vi "主流程.vi"() -> ()   [LabVIEW 2016]
panel:
  out "通讯包字符串":string
  out "列表选择":T1(ring)
  out "枚举":T2(ring)
  out "数据输出":string
  in  "IP":string
  in  "远程端口或服务名称":u16
  in  "停止 2":bool
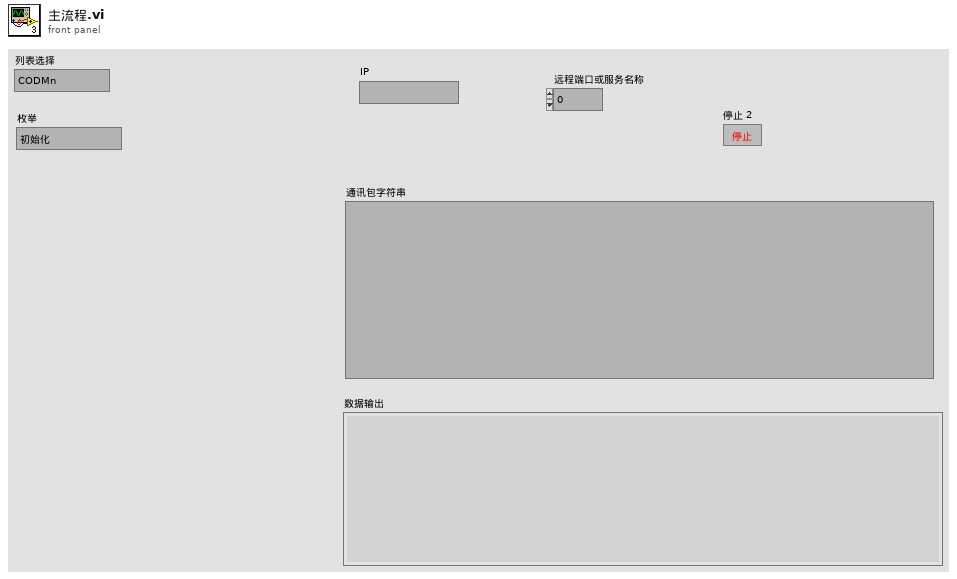
[diagram p1: front panel]
types:
  T1 = enum16{"CODMn", "CODMn空白核查", "CODMn标样核查", "氨氮", "氨氮空白核查", "氨氮标样核查", "多参数", "多参标样核查", "总磷", "总磷空白核查", "总磷标样核查", "总氮", "总氮空白核查", "总氮标样核查"}
  T2 = enum16{"初始化", "打开连接", "表格比对", "发送数据", "读取数据", "数据发送成功", "数据发送失败"}
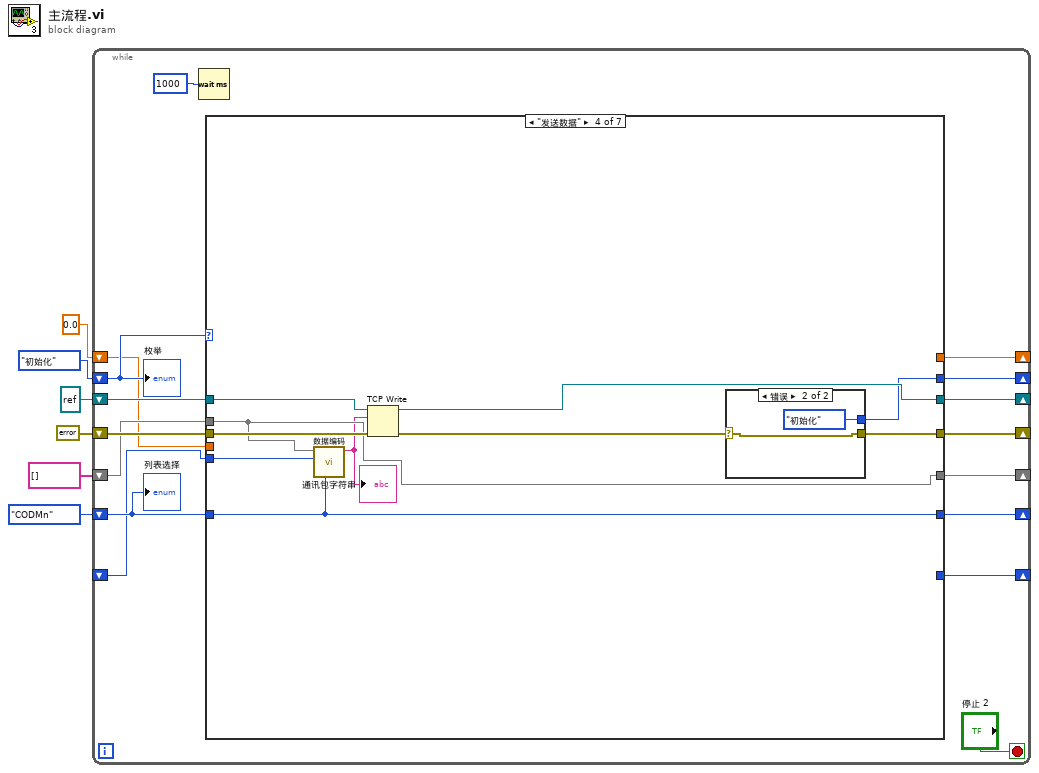
[diagram p0: block diagram]
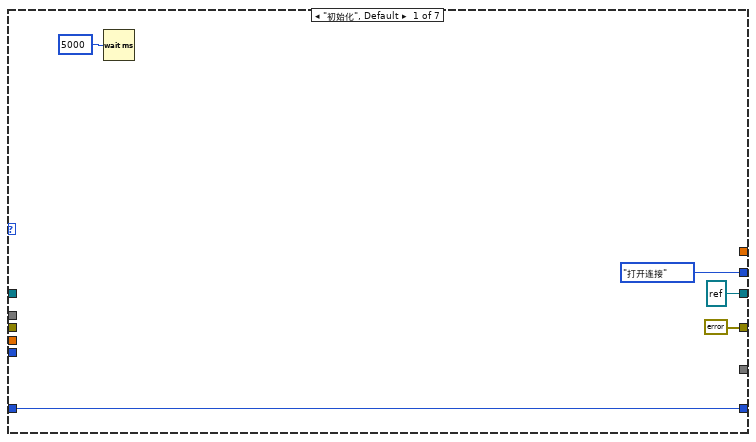
[diagram p2: hidden frame]
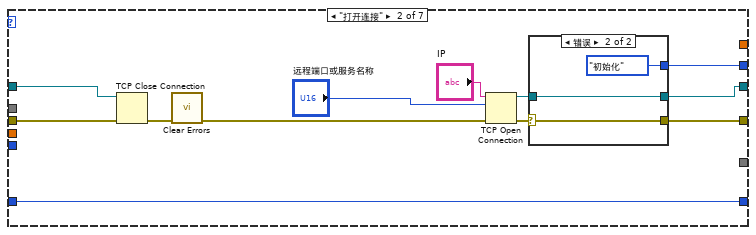
[diagram p3: hidden frame]
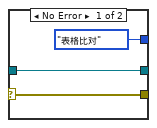
[diagram p4: hidden frame]
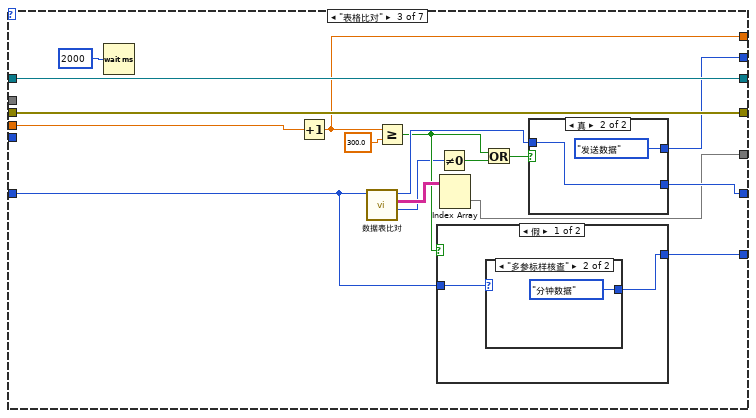
[diagram p5: hidden frame]
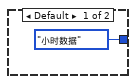
[diagram p6: hidden frame]
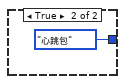
[diagram p7: hidden frame]
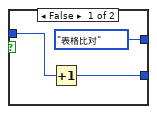
[diagram p8: hidden frame]
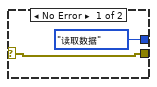
[diagram p9: hidden frame]
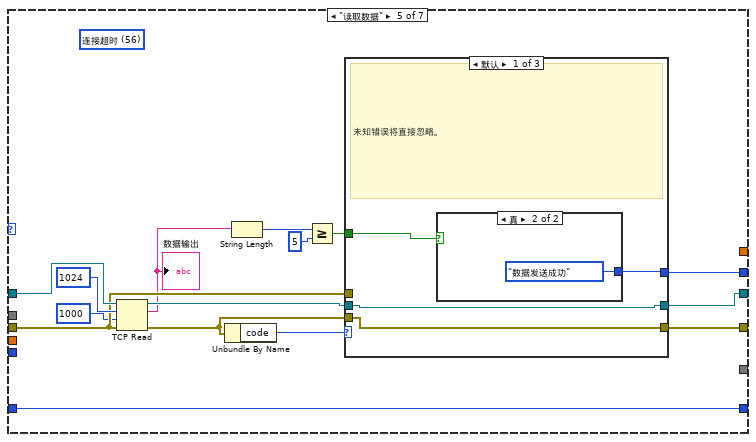
[diagram p10: hidden frame]
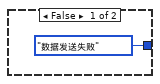
[diagram p11: hidden frame]
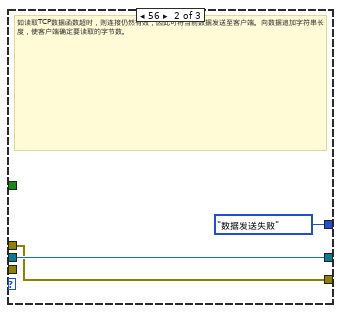
[diagram p12: hidden frame]
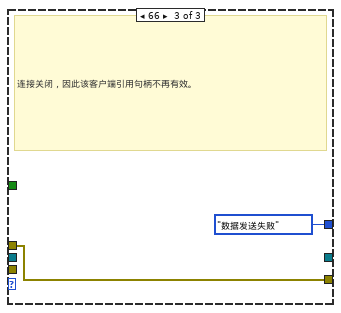
[diagram p13: hidden frame]
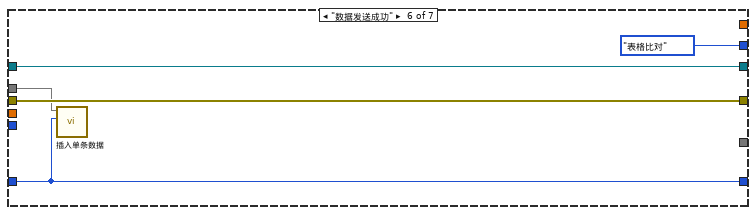
[diagram p14: hidden frame]
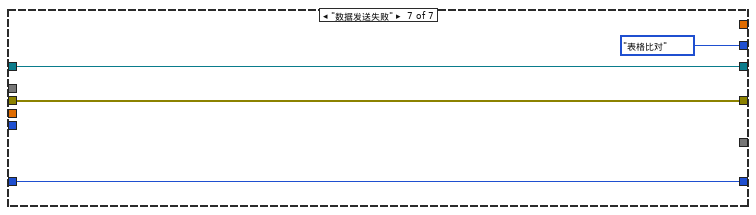
[diagram p15: hidden frame]
diagram:
  n1 = while {
    shift-right: [w21] -> _
    shift-left: T2."初始化" ("枚举") -> [w22]
    shift-right: [w20] -> _
    shift-left: refnum<k5> refnum ("connection ID") -> [w18]
    shift-right: [w19] -> _
    shift-left: errorcluster {"status"=FALSE, "code"=0, "source"=""} ("error out") -> [w17]
    shift-right: [w14] -> _
    shift-left: T1."CODMn" ("列表选择") -> [w15]
    shift-right: [w13] -> _
    shift-left: string[] [] ("待发送数据") -> [w12]
    shift-right: [w9] -> _
    shift-left: 0.0 -> [w10]
    shift-right: [w8] -> _
    shift-left: _ -> [w7]
    stop <- "停止 2" stop-if-true
    n2 = Wait (ms)(milliseconds to wait=u32 1000 ("等待时间（毫秒）")) -> ()  [unwired: 1 out]
    n3 = case shown="\"发送数据\"" w22 {
      tunnel: [T2."打开连接" ("枚举") w39 w58 w76 w88 T2."表格比对" ("枚举") T2."表格比对" ("枚举")] -> w21
      tunnel: [refnum<k5> refnum ("connection ID") w29 w62 w80 w98 w117 w121] -> w20
      tunnel: [errorcluster {"status"=FALSE, "code"=0, "source"=""} ("error out") w31 w61 w75 w96 w116 w120] -> w19
      tunnel: w18 -> [_ w35 w62 w82 w101 w117 w121]
      tunnel: w17 -> [_ w34 w61 w81 w97 w116 w120]
      tunnel: w15 -> [w24 w28 w46 w73 w89 w113 w118]
      tunnel: [w24 w28 w60 w73 w89 w113 w118] -> w14
      tunnel: [_ _ w50 w79 _ _ _] -> w13
      tunnel: w12 -> [_ _ _ w79 _ w114 _]
      tunnel: w10 -> [_ _ w55 _ _ _ _]
      tunnel: [_ _ w54 _ _ _ _] -> w9
      tunnel: [_ _ w48 _ _ _ _] -> w8
      tunnel: w7 -> [_ _ _ w74 _ _ _]
      frame "初始化", Default {
        n4 = Wait (ms)(milliseconds to wait=u32 5000 ("等待时间（毫秒）")) -> ()  [unwired: 1 out]
      }
      frame "打开连接" {
        n5 = TCP Close Connection(connection ID=w35, error in (no error)=w34) -> (error out=w33:errorcluster)  [unwired: 1 in, 1 out]
        n6 = call <vilib>:"Clear Errors.vi"("error in (no error)"=w33) -> ("error out"=w32:errorcluster)  [unwired: 5 in, 1 out]
        n7 = TCP Open Connection(address="IP", remote port or service name="远程端口或服务名称", error in (no error)=w32) -> (connection ID=w30:refnum<k5>, error out=w36:errorcluster)  [unwired: 2 in]
        n8 = case shown="错误" w36 {
          selector: w36 -> [w40 w44]
          tunnel: [T2."表格比对" ("枚举") T2."初始化" ("枚举")] -> w39
          tunnel: [w40 w44] -> w31
          tunnel: w30 -> [w41 w43]
          tunnel: [w41 w43] -> w29
          frame No Error {
          }
          frame Error {
          }
        }
      }
      frame "表格比对" {
        n9 = Wait (ms)(milliseconds to wait=u32 2000 ("等待时间（毫秒）")) -> ()  [unwired: 1 out]
        n10 = Increment(x=w55) -> (x+1=w54:dbl)
        n11 = call "数据表比对.vi"("列表输入"=w46) -> ("待发送条数"=w47:i32, "待发送数据"=w57:string[][], "列表输出"=w59:T1)  [unwired: 7 in, 1 out]
        n12 = Greater Or Equal?(x=w54, y=300.0) -> (x >= y?=w49:bool)
        n13 = case shown="假" w49 {
          tunnel: [w64 enum16{"心跳包", "分钟数据", "小时数据"}."心跳包" ("发送数据类型")] -> w48
          tunnel: w46 -> [w63 _]
          frame False {
            n14 = case shown="\"多参标样核查\"" w63 {
              tunnel: [enum16{"心跳包", "分钟数据", "小时数据"}."小时数据" ("发送数据类型") enum16{"心跳包", "分钟数据", "小时数据"}."分钟数据" ("发送数据类型")] -> w64
              frame Default {
              }
              frame "多参标样核查" {
              }
            }
          }
          frame True {
          }
        }
        n15 = Not Equal To 0?(x=w47) -> (x != 0?=w51:bool)
        n16 = Index Array(array=w57) -> (element=w50:string[])  [unwired: 2 in]
        n17 = Or(x=w49, y=w51) -> (x .or. y?=w52:bool)
        n18 = case shown="真" w52 {
          tunnel: [w69 w72] -> w60
          tunnel: w59 -> [w70 w72]
          tunnel: [T2."表格比对" ("枚举") T2."发送数据" ("枚举")] -> w58
          frame False {
            n19 = Increment(x=w70) -> (x+1=w69:T1)
          }
          frame True {
          }
        }
      }
      frame "发送数据" {
        n20 = call "数据编码.vi"("列表选择"=w73, "发送数据类型"=w74, "待发送数据"=w79) -> ("通讯包字符串"=w78:string)  [unwired: 7 in, 1 out]
        "通讯包字符串" <- w78
        n21 = TCP Write(connection ID=w82, data in=w78, error in (no error)=w81) -> (connection ID out=w80:refnum<k5>, error out=w77:errorcluster)  [unwired: 1 in, 1 out]
        n22 = case shown="错误" w77 {
          selector: w77 -> [w83 w85]
          tunnel: [T2."读取数据" ("枚举") T2."初始化" ("枚举")] -> w76
          tunnel: [w83 w85] -> w75
          frame No Error {
          }
          frame Error {
          }
        }
      }
      frame "读取数据" {
        (unwired) 56 items=["无错误", "参数错误", "内存已满", "超出区域", "文件结束", "文件已打开", "一般文件IO错误", "未找到文件", "文件权限错误", "磁盘已满", "路径副本", "打开过多文件", "未启用", "未找到资源文件", "无法添加资源", "未找到资源", "未找到图像", "图像内存错误", "画笔不存在", "配置错误类型", "配置未找到解析段", "配置解析错误", "配置内存错误", "错误外部代码格式", "错误外部代码偏移量", "外部代码不存在", "空窗口", "销毁窗口错误", "空菜单", "打印已中止", "错误打印记录", "打印驱动程序错误", "打印时窗口错误", "打印时内存错误", "打印对话框错误", "一般打印错误", "无效设备引用句柄", "设备未找到", "设备参数错误", "设备单位错误", "无法打开设备", "设备调用已中止", "一般错误", "用户已取消", "对象ID过低", "对象ID过高", "对象不在堆中", "未知的堆", "错误DefProc ID", "DefProc不在表格中", "范围外信息", "空方法", "未知信息", "不支持管理器调用", "错误地址", "连接过程中", "连接超时", "连接过程中", "不支持网络属性", "网络错误", "正在使用的地址", "系统缺少内存", "连接已中止", "连接已拒绝", "连接未建立", "连接已建立", "连接已关闭", "初始化错误（交互应用程序管理器）", "错误事件发生", "等待无约束事件发生处理程序", "事件发生队列溢出", "错误路径", "未发出信号量", "未识别类型（交互应用程序管理器）"] ("1st Error to Convert")
        n23 = TCP Read(connection ID=w101, bytes to read=1024 ("读取的字节"), error in (no error)=w97, 9:1000 ("超时毫秒(25000)")) -> (connection ID out=w99:refnum<k5>, data out=w87:string, error out=w95:errorcluster)  [unwired: 1 in]
        "数据输出" <- w87
        n24 = Unbundle By Name(w95) -> ("code"=w94:i32)
        n25 = String Length(string=w87) -> (length=w92:i32)
        n26 = Greater Or Equal?(x=w92, y=5) -> (x >= y?=w90:bool)
        n27 = case shown="默认" w94 {
          tunnel: w95 -> [w105 _ _]
          tunnel: [w105 w109 w112] -> w96
          tunnel: w97 -> [_ w109 w112]
          tunnel: w99 -> [w104 w110 _]
          tunnel: [w104 w110 _] -> w98
          tunnel: w90 -> [w103 _ _]
          tunnel: [w102 T2."数据发送失败" ("枚举") T2."数据发送失败" ("枚举")] -> w88
          frame Default {
            # "未知错误将直接忽略。"
            n28 = case shown="真" w103 {
              tunnel: [T2."数据发送失败" ("枚举") T2."数据发送成功" ("枚举")] -> w102
              frame False {
              }
              frame True {
              }
            }
          }
          frame 56 {
            # "如读取TCP数据函数超时，则连接仍然有效，因此可将当前数据发送至客户端。向数据追加字符串长度，使客户端确定要读取的字节数。"
          }
          frame 66 {
            # "连接关闭，因此该客户端引用句柄不再有效。"
          }
        }
      }
      frame "数据发送成功" {
        n29 = call "插入单条数据.vi"("table"=w113, "插入数据"=w114) -> ()  [unwired: 8 in, 2 out]
      }
      frame "数据发送失败" {
      }
    }
    "枚举" <- w22
    "列表选择" <- w15
  }
